vi "LQR_v1.vi"() -> ()   [LabVIEW 2018]
uses:
  <vilib>/imath/engines/lvmath2/RunTimeEngine/IndexRead/NIMS M(S,S).vi
  <instcachedir>/0/NIMS M(S,S)_AC51E74150A542F7991B9634C66F3096.lvgen/NIMS M(S,S)_AC51E74150A542F7991B9634C66F3096_000.vi
  <vilib>/imath/engines/lvmath2/RunTimeEngine/IndexRead/NIMS V(S).vi
  <instcachedir>/0/NIMS V(S)_0488751826AF41519A22953C041130DC.lvgen/NIMS V(S)_0488751826AF41519A22953C041130DC_000.vi
  <vilib>/imath/engines/lvmath2/RunTimeEngine/IndexReplace/NIMS M(S,S)=S.vi
  <instcachedir>/0/NIMS M(S,S)=S_5DAF17B45D8A4C8588C7CF468644990A.lvgen/NIMS M(S,S)=S_5DAF17B45D8A4C8588C7CF468644990A_000.vi
  <vilib>/imath/engines/lvmath2/RunTimeEngine/ErrorHandling/NIMS_Create Error From Enums.vi
  <vilib>/imath/engines/lvmath/Plug In/Control Design/BuiltInFunctions/ss/NIMS_CD_ss(A,B,C,D).vi
  <vilib>/imath/engines/lvmath2/RunTimeEngine/NodeEndStatement/NIMS_NodeEndStatement_Output.vi
  <instcachedir>/0/NIMS_NodeEndStatement_Output_53EC0D466D134D7ABD903AC30B43404B.lvgen/NIMS_NodeEndStatement_Output_53EC0D466D134D7ABD903AC30B43404B_012.vi
  <vilib>/imath/engines/lvmath2/RunTimeEngine/ErrorHandling/NIMS_Finalize Error.vi
  <vilib>/addons/Control Design/_State Feedback Control/State Feedback Control.llb/State Feedback Control SubVis/cd_Linear Quadratic Regulator.vi
  <vilib>/addons/Control Design/_State Feedback Control/NI_CD_State Feedback Control.lvlib
panel:
  out "Optimal Gain (K)":dbl[][](array[numeric]) format="%.2f"
  in  "R":dbl[][](array[numeric]) format="%.2f"
  in  "Q":dbl[][](array[numeric]) format="%.2f"
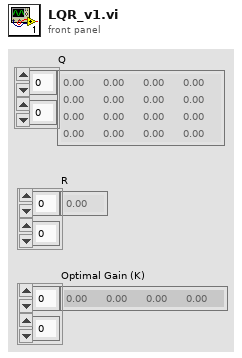
[diagram p1: front panel]
types:
  T1 = typedef "NI_LinSys_Model Typedefs.lvlib/CD State Space Model (MIMO).ctl" = cluster{"properties":T2, "A":dbl[][], "B":dbl[][], "C":dbl[][], "D":dbl[][], "StateNames":string[], "Transport Delay":dbl[][]}
  T2 = typedef "NI_LinSys_Model Typedefs.lvlib/CD General Elements.ctl" = cluster{"Model name":string, "Input names":string[], "Output names":string[], "Input Delays":dbl[], "Output Delays":dbl[], "Sampling Time":dbl, "Notes":string}
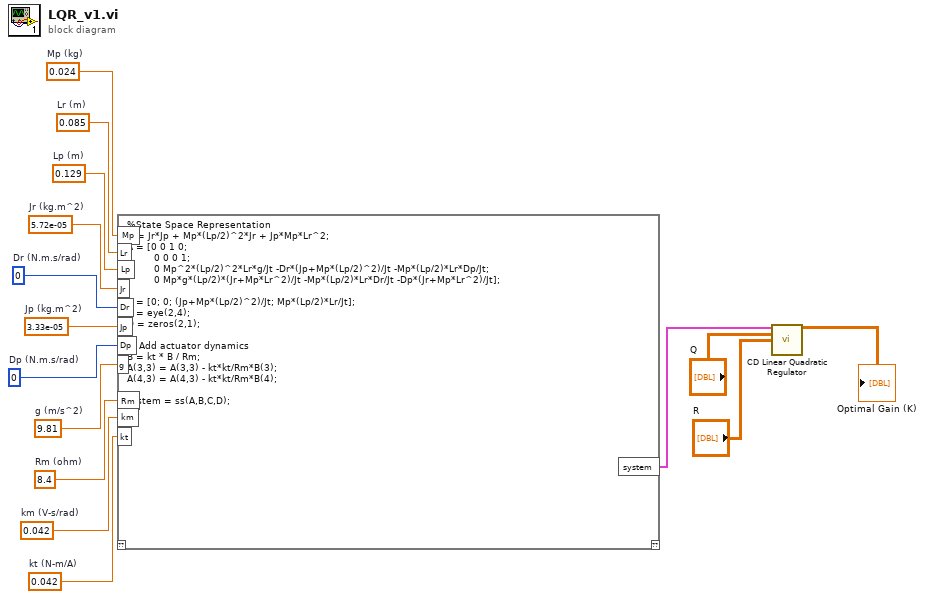
[diagram p0: block diagram]
diagram:
  w5 = 0.042  # kt (N-m/A)
  w6 = 0.042  # km (V-s/rad)
  w7 = 8.4  # Rm (ohm)
  w8 = 9.81  # g (m/s^2)
  w9 = 0  # Dp (N.m.s/rad)
  w10 = 3.33e-05  # Jp (kg.m^2)
  w11 = 0  # Dr (N.m.s/rad)
  w13 = 0.129  # Lp (m)
  w12 = 5.72e-05  # Jr (kg.m^2)
  w14 = 0.085  # Lr (m)
  w15 = 0.024  # Mp (kg)
  n1 = mathscript code="%State Space Representation\nJt = Jr*Jp + Mp*(Lp/2)^2*Jr + Jp*Mp*Lr^2;\nA = [0 0 1 0;\n         0 0 0 1;\n         0 Mp^2*(Lp/2)^2*Lr*g/Jt -Dr*(Jp+Mp*(Lp/2)^2)/Jt -Mp*(Lp/2)*Lr*Dp/Jt;\n         0 Mp*g*(Lp/2)*(Jr+Mp*Lr^2)/Jt -Mp*(Lp/2)*Lr*Dr/Jt -Dp*(Jr+Mp*Lr^2)/Jt];\n\nB = [0; 0; (Jp+Mp*(Lp/2)^2)/Jt; Mp*(Lp/2)*Lr/Jt];\nC = eye(2,4);\nD = zeros(2,1);\n\n% Add actuator dynamics\nB = kt * B / Rm;\nA(3,3) = A(3,3) - kt*kt/Rm*B(3);\nA(4,3) = A(4,3) - kt*kt/Rm*B(4);\n\nsystem = ss(A,B,C,D);"("Mp"=w15, "Lr"=w14, "Lp"=w13, "Jr"=w12, "Dr"=w11, "Jp"=w10, "Dp"=w9, "g"=w8, "Rm"=w7, "km"=w6, "kt"=w5) -> ("system"=w4:T1)  [unwired: 1 in, 1 out]
  n2 = call-poly <vilib>:"CD Linear Quadratic Regulator.vi"("State-Space Model"=w4, "Q"="Q", "R"="R") -> ("Optimal Gain (K)"=→"Optimal Gain (K)":dbl[][])  [unwired: 9 in, 3 out]
